vi "TEMPLATE_Constructor.vi"(8 "Error In":errorcluster) -> (0 "Error Out":errorcluster, 3 "QObject Out":refnum<class "QObject.lvclass">)   [LabVIEW 2013, in "Template.lvlib" / "QObject.lvclass"]
uses:
  QObject.lvclass
  QObject.lvclass/QObject.ctl
  LQWidgetEngine/LQWidgetEngine.lvclass
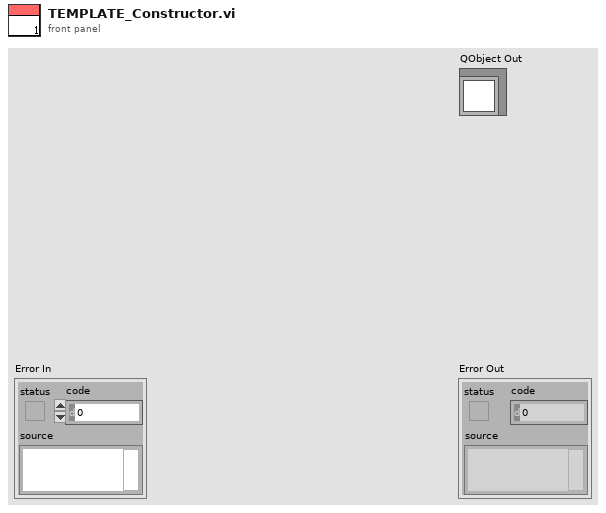
[diagram p1: front panel]
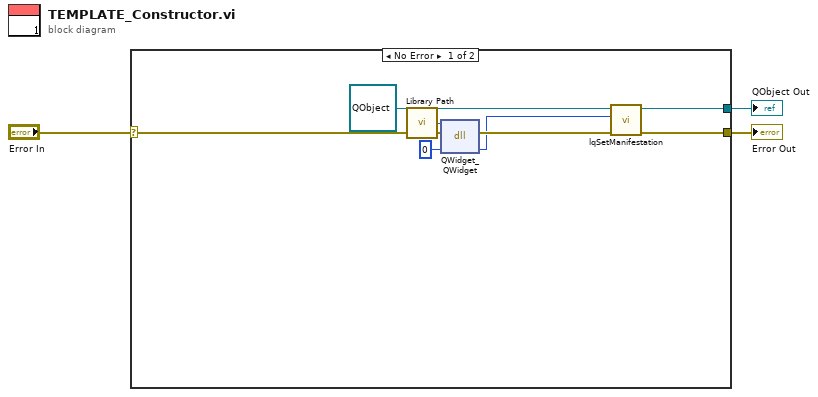
[diagram p0: block diagram]
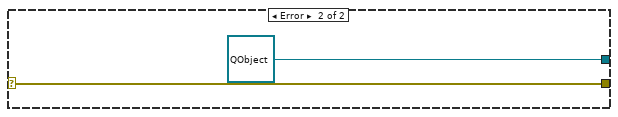
[diagram p2: hidden frame]
diagram:
  n1 = case shown="No Error" "Error In" {
    selector: "Error In" -> [w11 w13]
    tunnel: [w7 w13] -> w2
    tunnel: [w9 refnum<class "QObject.lvclass"> refnum ("QObject")] -> w1
    frame No Error {
      n2 = call "Library Path.vi"() -> ("Library Path"=w4:path)
      n3 = dll-call lib="?" fn="QWidget_QWidget"(path in=w4, error in=w11, "obj"=u32 0) -> (error out=w8:errorcluster, "obj"=w6:u32)  [unwired: 2 in, 1 out]
      n4 = call "lqSetManifestation.vi"("error in (no error)"=w8, "Manifestation"=w6, "QObject in"=refnum<class "QObject.lvclass"> refnum ("QObject")) -> ("error out"=w7:errorcluster, "QObject out"=w9:refnum<class "QObject.lvclass">)  [unwired: 7 in]
    }
    frame Error {
    }
  }
  "Error Out" <- w2
  "QObject Out" <- w1
